vi "Calibrate Ruler.vi"() -> ()   [LabVIEW 2014]
uses:
  <vilib>/vision/NI_Vision_Development_Module.lvlib
  <vilib>/Platform/NI_3dgraph.lvlib
  <vilib>/Analysis/NI_AALBase.lvlib
panel:
  out "nm / pixel":dbl=65.359477124183
  out "size(s) 2":i32
  in  "most value":i32=147
  out "distance 2":i32[](array[numeric])
  out "Histogram Graph":T1(graph)
  out "distance":i32[](array[numeric])
  out "index":i32[][](array[numeric])
  out "min value":u8[][](array[numeric])
  in  "# line":i32
  out "Numeric":i32
  in  "3D Curve":refnum<k7>(container)
  out "size(s)":i32[](array[numeric])
  out "x vectors 2":i32[](array[numeric])
  out "y vectors 2":i32[](array[numeric])
  out "x vectors":i32[](array[numeric])
  out "y vectors":i32[](array[numeric])
  out "width (pixel)":i32
  out "height (pixel)":i32
  in  "Optional Rectangle":i32[](array[numeric])=[1300, 0]
  out "Image 2":T2(plugin-control)
  out "Image":T2(plugin-control)
  in  "File Path":path
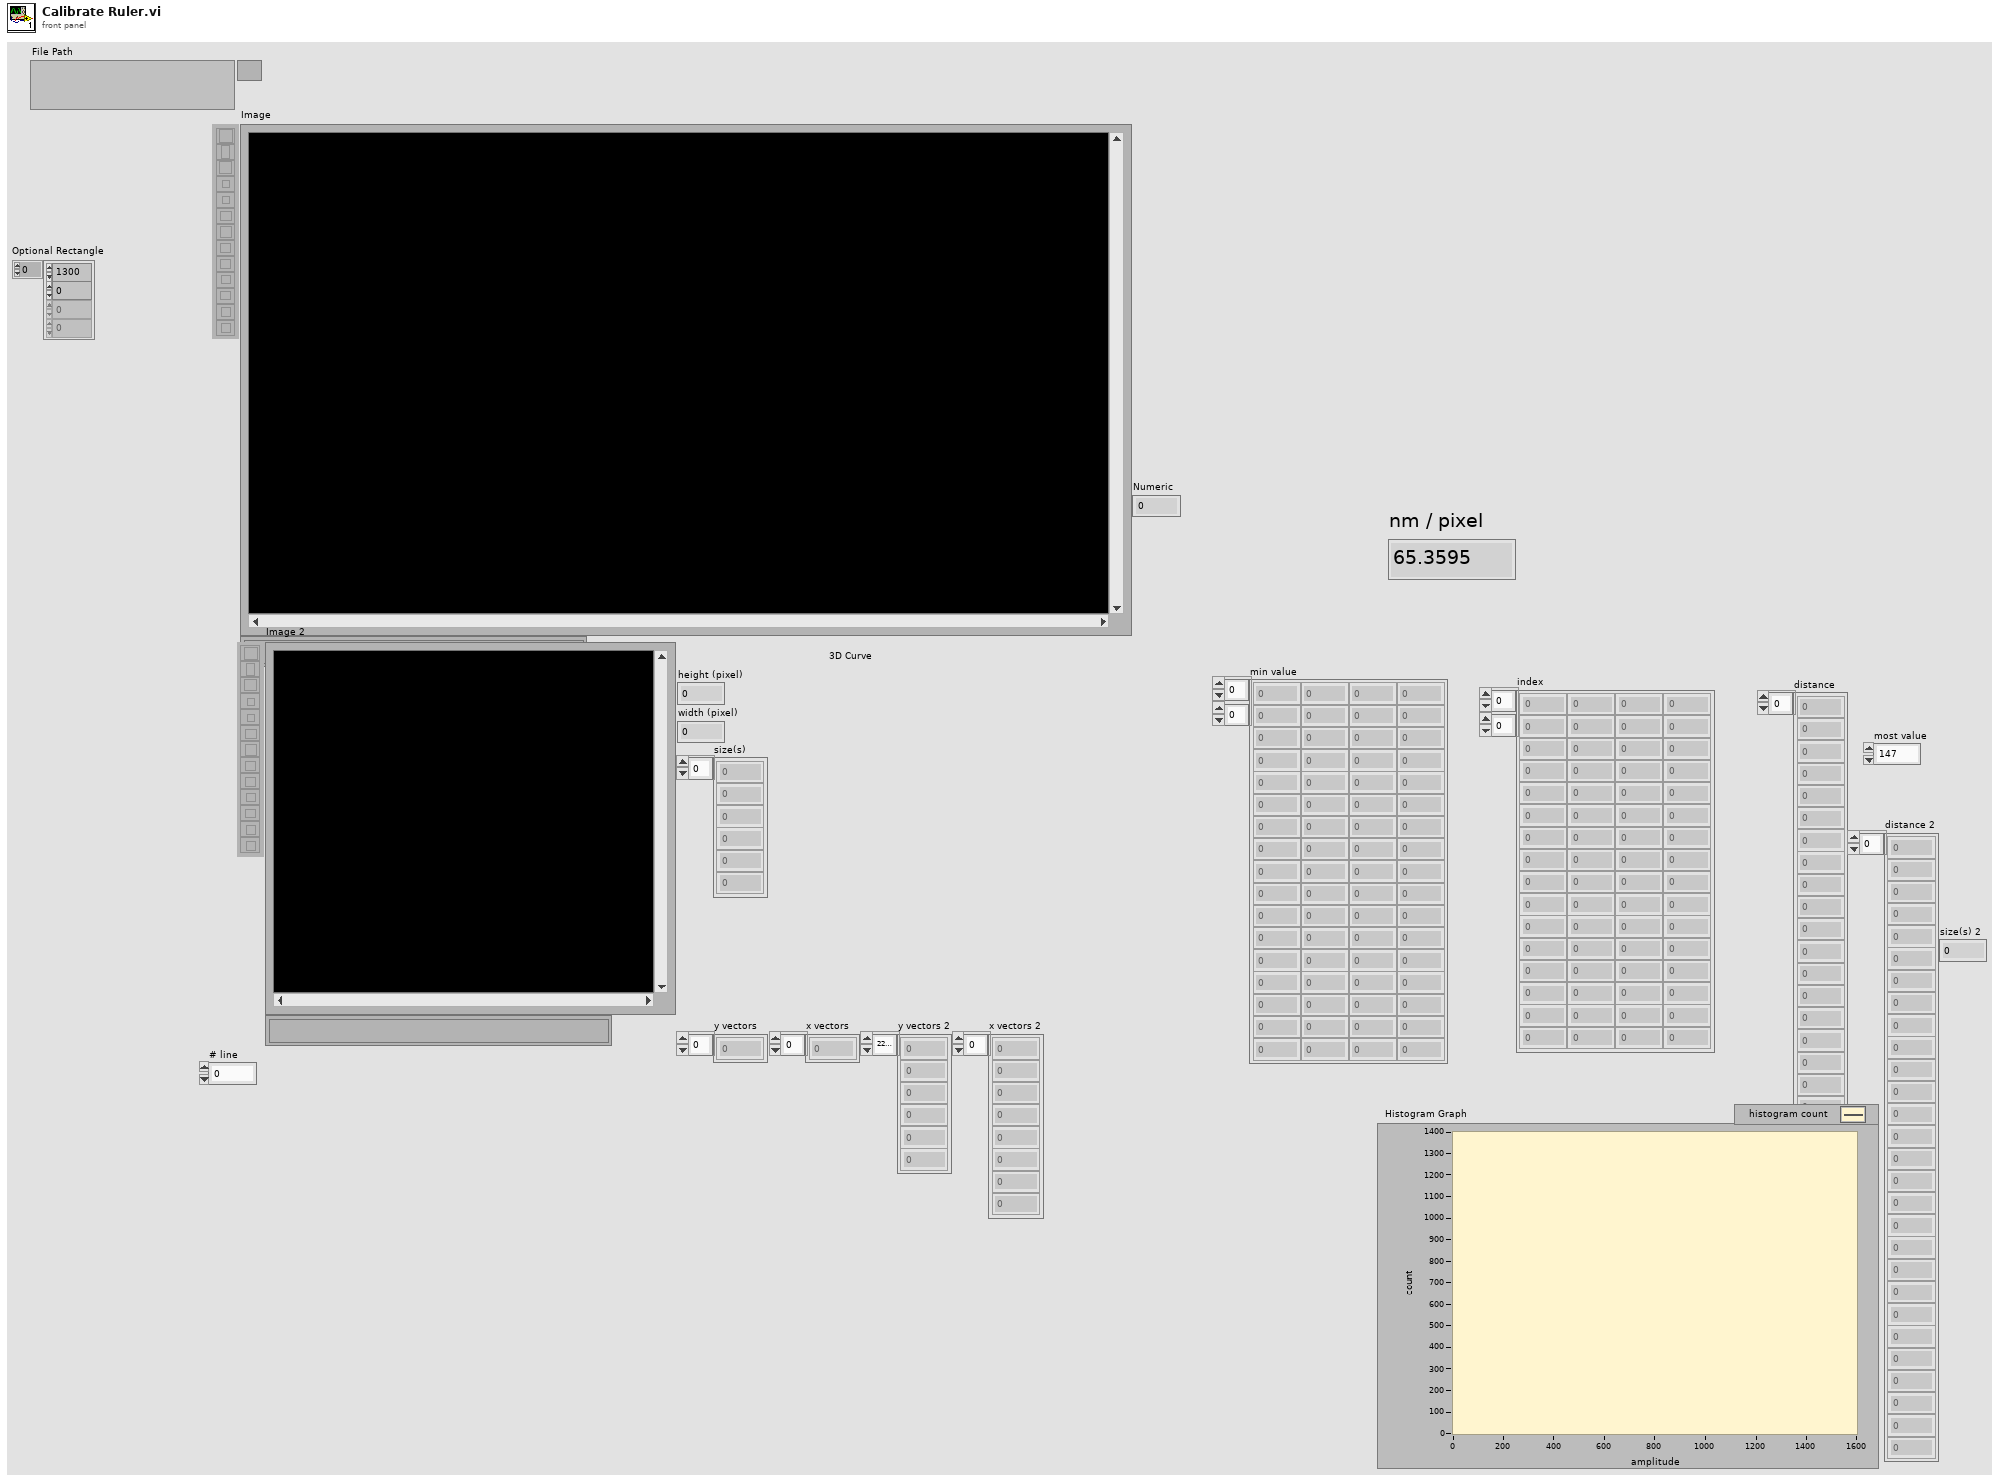
[diagram p1: front panel]
types:
  T1 = cluster{"X Values":dbl[], "Histogram: h(x)":i32[]}
  T2 = typedef "IMAQ Image.ctl" = refnum<image>
  T3 = typedef "Image Type" = u32
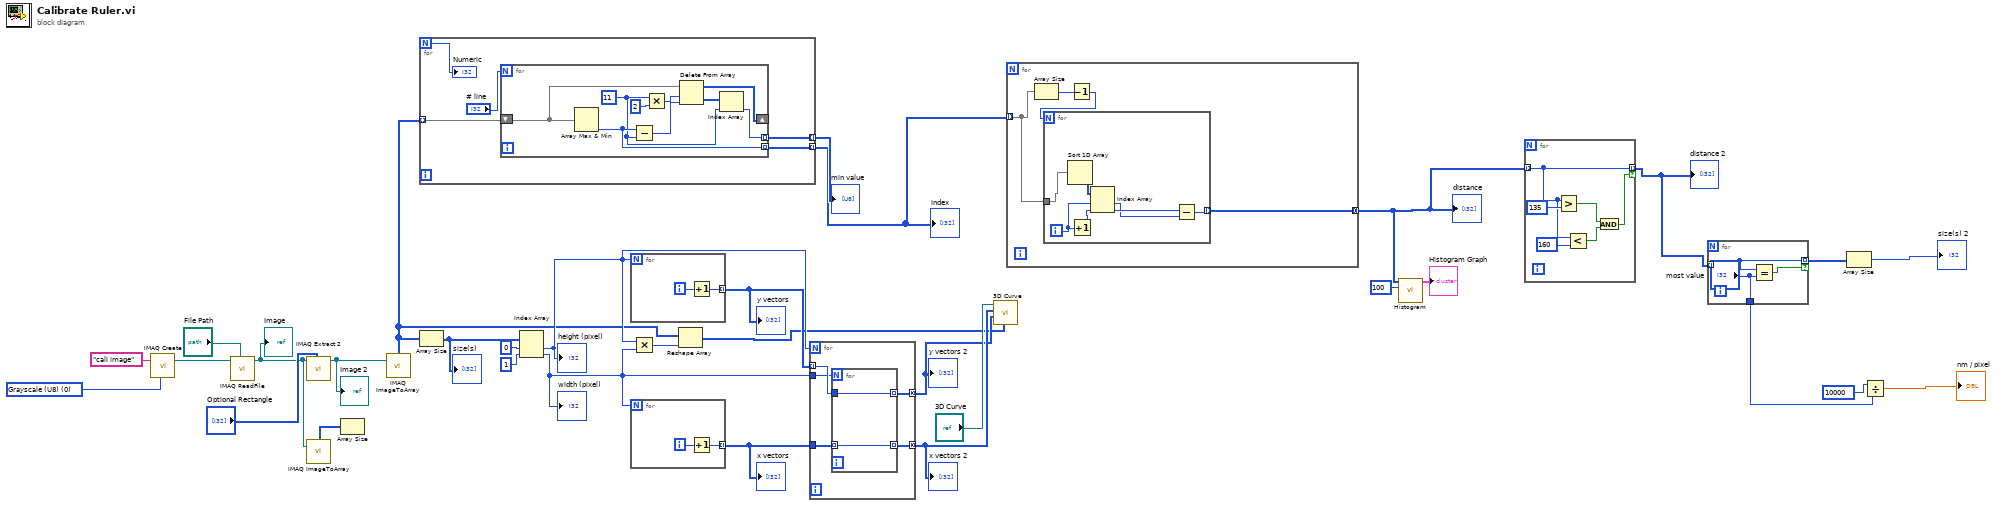
[diagram p0: block diagram]
diagram:
  w30 = T3 0 items=["Grayscale (U8)", "Grayscale (I16)", "Grayscale (SGL)", "Complex (CSG)", "RGB (U32)", "HSL (U32)", "RGB (U64)", "Grayscale (U16)"] ("Image Type")
  n1 = call "IMAQ Create"("Image Name"="cali image", "Image Type"=w30) -> ("New Image"=w29:T2)  [unwired: 3 in, 1 out]
  n2 = call "IMAQ ReadFile"("File Path"="File Path", "Image"=w29) -> ("Image Out"=w26:T2)  [unwired: 5 in, 4 out]
  "Image" <- w26
  n3 = call "IMAQ Extract 2"("Optional Rectangle"="Optional Rectangle", "Image Src"=w26) -> ("Image Dst Out"=w18:T2)  [unwired: 8 in, 1 out]
  "Image 2" <- w18
  n4 = call "IMAQ ImageToArray"("Image"=w26) -> ("Image Pixels (U8)"=w25:u8[][])  [unwired: 3 in, 4 out]
  n5 = Array Size(array=w25) -> ()  [unwired: 1 out]
  n6 = call "IMAQ ImageToArray"("Image"=w18) -> ("Image Pixels (U8)"=w12:u8[][])  [unwired: 3 in, 4 out]
  n7 = for {
    N -> [w37]
    tunnel: w12 -> [w36] mode=indexing
    tunnel: [w34] -> w11 mode=indexing
    tunnel: [w33] -> w10 mode=indexing
    n8 = for {
      N: "# line" -> [_]
      shift-right: [w45] -> _
      shift-left: w36 -> [w46]
      tunnel: [w43] -> w34 mode=indexing
      tunnel: [w42] -> w33 mode=indexing
      w38 = 11 ("y")
      n9 = Array Max & Min(array=w46) -> (min index (indices)=w42:i32)  [unwired: 3 out]
      n10 = Subtract(x=w42, y=w38) -> (x-y=w41:i32)
      n11 = Multiply(x=w38, y=2 ("length")) -> (x*y=w39:i32)
      n12 = Delete From Array(array=w46, length=w39, index=w41) -> (deleted portion=w44:u8[], array with subset deleted=w45:u8[])
      n13 = Index Array(array=w44, index=w38) -> (element=w43:u8)
    }
    "Numeric" <- w37
  }
  "min value" <- w11
  "index" <- w10
  n14 = Array Size(array=w12) -> (size(s)=w22:i32[])
  "size(s)" <- w22
  n15 = Index Array(array=w22, index #1=0 ("index"), index #2=1 ("index")) -> (element #1=w20:i32, element #2=w19:i32)
  "height (pixel)" <- w20
  "width (pixel)" <- w19
  n16 = for {
    N: w20 -> [_]
    tunnel: [w47] -> w21 mode=indexing
    i -> [w48]
    n17 = Increment(x=w48) -> (x+1=w47:i32)
  }
  "y vectors" <- w21
  n18 = for {
    N: w19 -> [_]
    tunnel: [w49] -> w27 mode=indexing
    i -> [w50]
    n19 = Increment(x=w50) -> (x+1=w49:i32)
  }
  "x vectors" <- w27
  n20 = Multiply(x=w20, y=w19) -> (x*y=w17:i32)
  n21 = Reshape Array(w12, w17) -> (w13:u8[])
  n22 = for {
    N: w20 -> [_]
    tunnel: w27 -> [w55]
    tunnel: w21 -> [w54] mode=indexing
    tunnel: [w53] -> w15 mode=concatenating
    tunnel: [w52] -> w14 mode=concatenating
    tunnel: w19 -> [w51]
    n23 = for {
      N: w51 -> [_]
      tunnel: w55 -> [w57] mode=indexing
      tunnel: w54 -> [w56]
      tunnel: [w57] -> w53 mode=indexing
      tunnel: [w56] -> w52 mode=indexing
    }
  }
  "y vectors 2" <- w14
  "x vectors 2" <- w15
  n24 = call <vilib>:"3D Curve.vi"("z vector"=w13, "y vector"=w14, "x vector"=w15, "3D graph"="3D Curve") -> ()  [unwired: 6 in, 2 out]
  n25 = for {
    tunnel: w10 -> [w59] mode=indexing
    tunnel: [w58] -> w2 mode=concatenating
    n26 = Array Size(array=w59) -> (size(s)=w61:i32)
    n27 = Decrement(x=w61) -> (x-1=w60:i32)
    n28 = for {
      N: w60 -> [_]
      tunnel: w59 -> [w63]
      tunnel: [w64] -> w58 mode=indexing
      i -> [w68]
      n29 = Sort 1D Array(array=w63) -> (sorted array=w62:i32[])
      n30 = Increment(x=w68) -> (x+1=w67:i32)
      n31 = Index Array(array=w62, index #1=w68, index #2=w67) -> (element #1=w65:i32, element #2=w66:i32)
      n32 = Subtract(x=w66, y=w65) -> (x-y=w64:i32)
    }
  }
  "distance" <- w2
  n33 = call <vilib>:"Histogram.vi"("intervals"=100, "X"=w2) -> ("Histogram Graph"=→"Histogram Graph":T1)  [unwired: 6 in, 3 out]
  n34 = for {
    tunnel: w2 -> [w73] mode=indexing
    tunnel: [w73] -> w7 mode=indexing if=w69
    n35 = Greater?(x=w73, y=135) -> (0:w70:bool)
    n36 = Less?(x=w73, y=160) -> (x < y?=w71:bool)
    n37 = And(x=w70, y=w71) -> (x .and. y?=w69:bool)
  }
  "distance 2" <- w7
  n38 = for {
    tunnel: w7 -> [w77] mode=indexing
    tunnel: [w77] -> w6 mode=indexing if=w76
    tunnel: ["most value"] -> w1
    n39 = Equal?(x=w77, y="most value") -> (x = y?=w76:bool)
  }
  n40 = Array Size(array=w6) -> (size(s)=→"size(s) 2":i32)
  n41 = Divide(x=10000 ("y"), y=w1) -> (x/y=→"nm / pixel":dbl)
